vi "SetLabel.vi"(8 "error in (no error)":errorcluster, 10 "Label":string, 11 "DataProcessor in":refnum<class "DataProcessor.lvclass">) -> (0 "error out":errorcluster, 3 "DataProcessor out":refnum<class "DataProcessor.lvclass">)   [LabVIEW 2020, in "DataProcessor.lvlib" / "DataProcessor.lvclass"]
uses:
  DataProcessor.lvclass
  DataProcessor.lvclass/DataProcessor.ctl
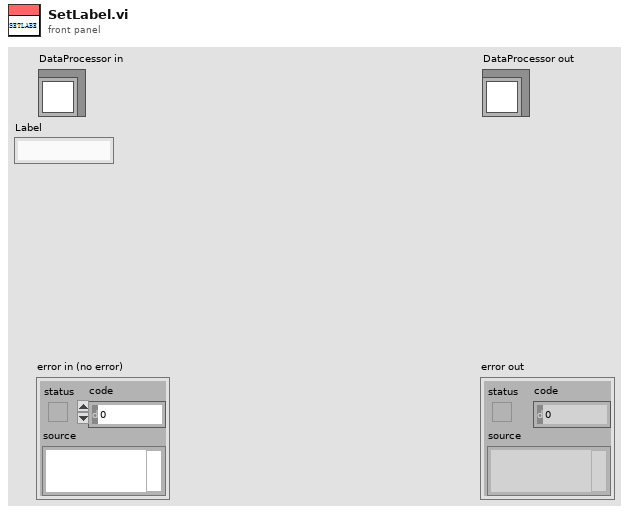
[diagram p1: front panel]
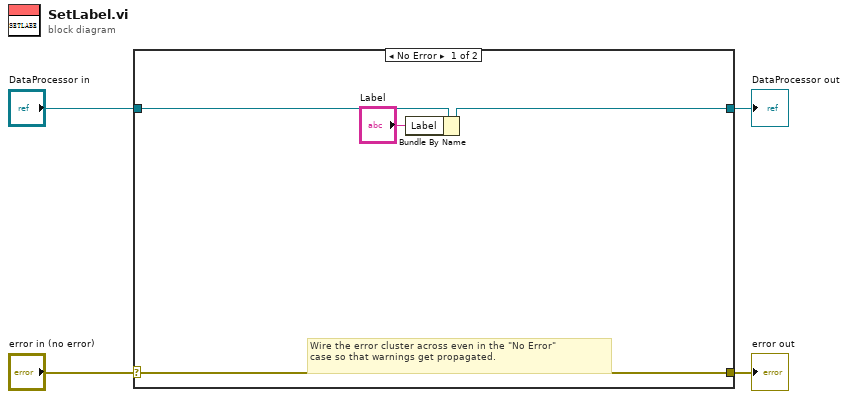
[diagram p0: block diagram]
diagram:
  n1 = case shown="No Error" "error in (no error)" {
    selector: "error in (no error)" -> [w7 w10]
    tunnel: [w7 w10] -> w3
    tunnel: [w6 w9] -> w1
    tunnel: "DataProcessor in" -> [w8 w9]
    frame No Error {
      # "Wire the error cluster across even in the \"No Error\"\ncase so that warnings get propagated."
      n2 = Bundle By Name(cluster=w8, "Label"="Label") -> (w6:refnum<class "DataProcessor.lvclass">)
    }
    frame Error {
    }
  }
  "error out" <- w3
  "DataProcessor out" <- w1
